vi "Recieve Status.vi"(8 "error in (no error)":errorcluster, 9 "Status offset":u64, 10 "Read config instead":bool, 11 "RP Communicator in":refnum<class "RP Communicator VISA.lvclass">) -> (0 "error out":errorcluster, 1 "Status response":u32=1 format="0x%x (%d)", 3 "RP Communicator out":refnum<class "RP Communicator VISA.lvclass">)   [LabVIEW 2015, in "RP Communicator VISA.lvclass"]
uses:
  RP Communicator VISA.lvclass
  RP Read Status VISA.vi
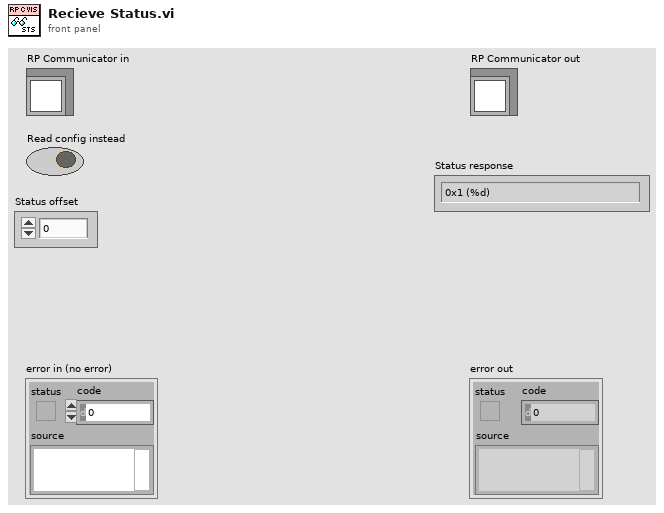
[diagram p1: front panel]
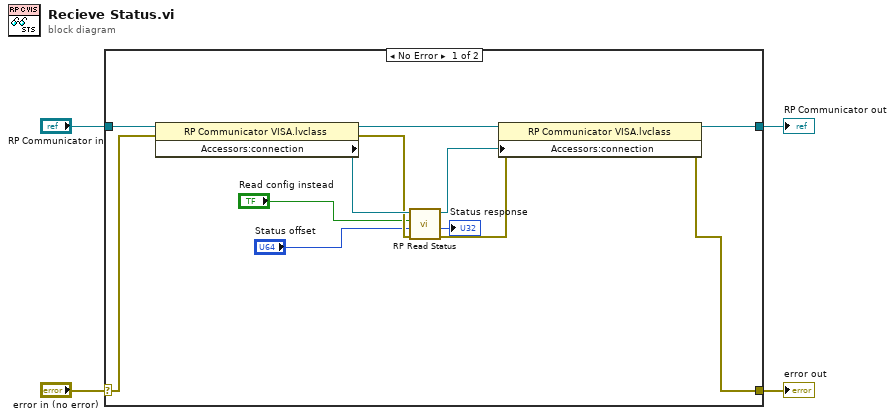
[diagram p0: block diagram]
diagram:
  n1 = case shown="No Error" "error in (no error)" {
    selector: "error in (no error)" -> [w8 w18]
    tunnel: [w10 w18] -> w3
    tunnel: [w13 w17] -> w1
    tunnel: "RP Communicator in" -> [w16 w17]
    frame No Error {
      n2 = property class="RP Communicator VISA.lvclass"(reference=w16, error in=w8) -> (reference out=w15:refnum<class "RP Communicator VISA.lvclass">, error out=w9:errorcluster, "Accessors:connection"=w14:refnum<visa-resource-name>)
      n3 = call-poly "RP Read Status.vi"("Error In"=w9, "Status offset"="Status offset", "Read config"="Read config instead", "VISA resource"=w14) -> ("Error Out"=w11:errorcluster, "Status response"=→"Status response":u32, "VISA resource out"=w12:refnum<visa-resource-name>)  [unwired: 5 in]
      n4 = property class="RP Communicator VISA.lvclass"(reference=w15, error in=w11, "Accessors:connection"=w12) -> (reference out=w13:refnum<class "RP Communicator VISA.lvclass">, error out=w10:errorcluster)
    }
    frame Error {
    }
  }
  "error out" <- w3
  "RP Communicator out" <- w1
